vi "Create Menus.vi"(6 "menu options":cluster{"open":bool, "save":bool, "view":bool}={"open"=TRUE, "save"=FALSE, "view"=FALSE}, 8 "error in (no error)":errorcluster, 11 "Application Data in":T1) -> (0 "error out":errorcluster, 3 "Application Data out":T1)   [LabVIEW 2017, in "DSF Core.lvlib"]
uses:
  DSF Core.lvlib
  Application Data.ctl
  <vilib>/NI/Memory Manager/Classes/Pointer/Pointer.lvclass
  Classes/Framework/Framework.lvclass
  Buffer Reader/Buffer Data.ctl
  Classes/Buffer/Buffer.lvclass
  Classes/Status/Status.lvclass
  Typedefs/DSF Data Type.ctl
  Typedefs/DSF Engine Channel Configuration.ctl
  Typedefs/DSF Settings Info.ctl
  Typedefs/DSF Byte Order.ctl
  Typedefs/DSF Engine Framework Configuration.ctl
  Typedefs/DSF Engine Plugin Configuration.ctl
  Typedefs/DSF Timing Info.ctl
  Typedefs/DSF Engine Plugin Thread Configuration.ctl
  Typedefs/DSF Engine Transfer Group Configuration.ctl
  Typedefs/DSF Direction.ctl
  Typedefs/DSF Engine Transfer Configuration.ctl
  Typedefs/DSF Timeout Behavior.ctl
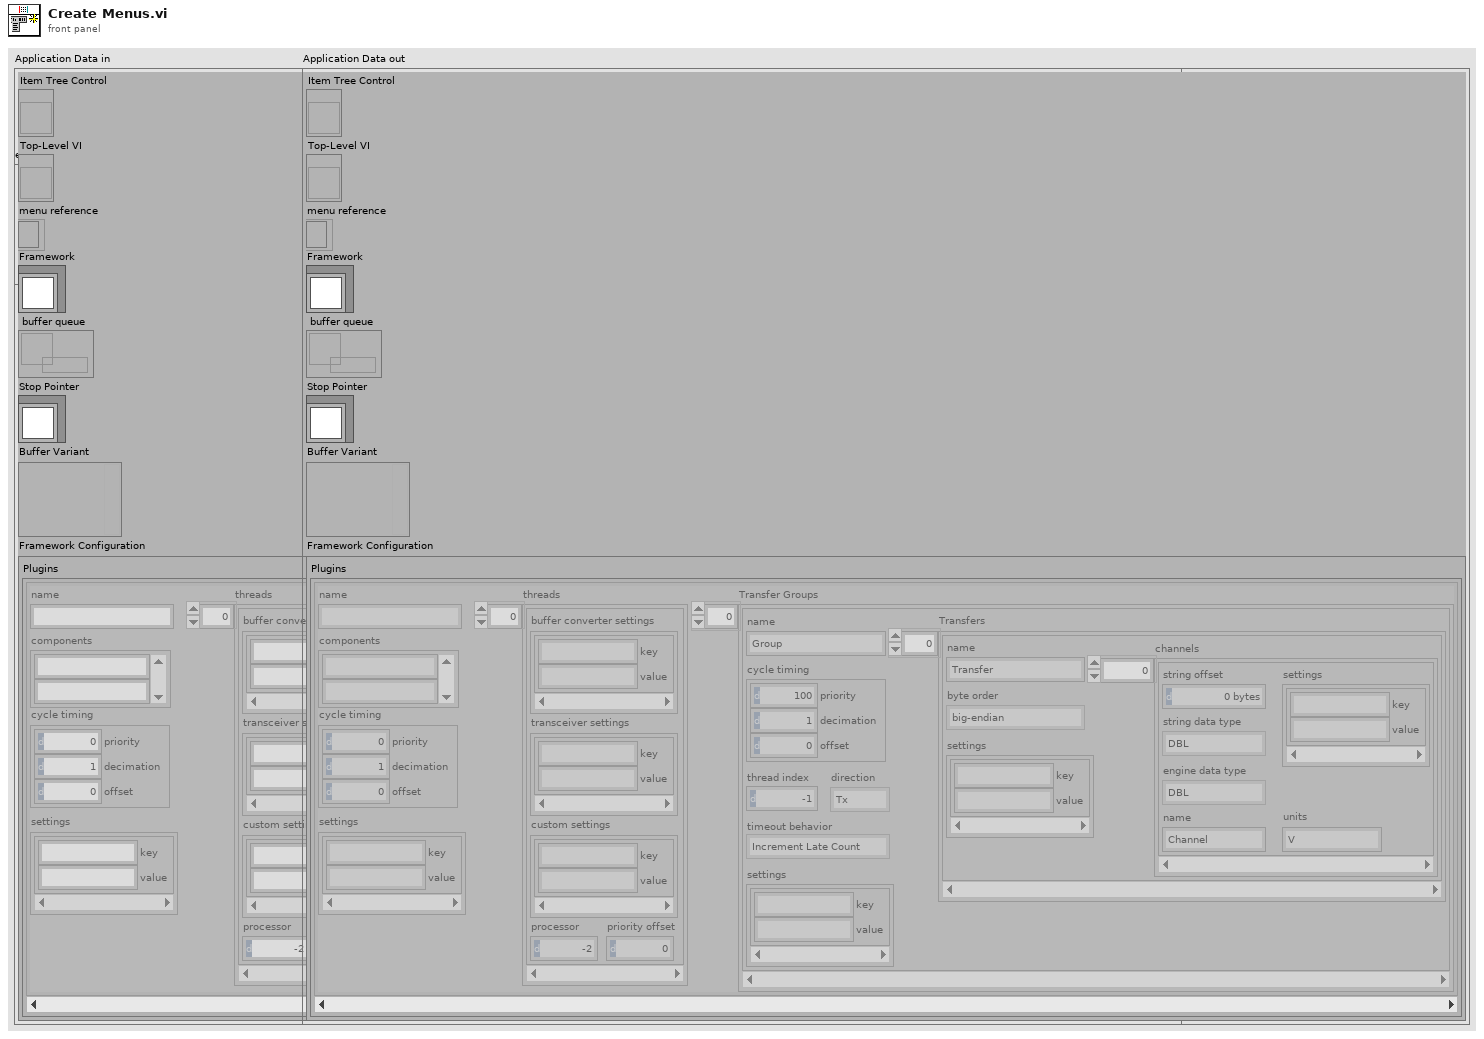
[diagram p1: front panel]
types:
  T1 = typedef "DSF Core.lvlib/Application Data.ctl" = cluster{"Item Tree Control":refnum<vi>, "Top-Level VI":refnum<vi>, "menu reference":refnum<k9>, "Framework":refnum<class "Framework.lvclass">, "buffer queue":refnum<queue>, "Stop Pointer":refnum<class "Pointer.lvclass">, "Buffer Variant":variant, "Framework Configuration":T2}
  T2 = typedef "DSF Core.lvlib/DSF Engine Framework Configuration.ctl" = cluster{"Plugins":T3[]}
  T3 = typedef "DSF Core.lvlib/DSF Engine Plugin Configuration.ctl" = cluster{"name":string, "components":string[], "cycle timing":T4, "threads":T5[], "Transfer Groups":T7[], "settings":T6}
  T4 = typedef "DSF Core.lvlib/DSF Timing Info.ctl" = cluster{"priority":u64, "decimation":u64, "offset":u64}
  T5 = typedef "DSF Core.lvlib/DSF Engine Plugin Thread Configuration.ctl" = cluster{"buffer converter settings":T6, "transceiver settings":T6, "custom settings":T6, "processor":i32, "priority offset":i16}
  T6 = typedef "DSF Core.lvlib/DSF Settings Info.ctl" = cluster{"key":string, "value":string}[]
  T7 = typedef "DSF Core.lvlib/DSF Engine Transfer Group Configuration.ctl" = cluster{"name":string, "direction":T8, "cycle timing":T4, "thread index":i32, "settings":T6, "Transfers":T9[], "timeout behavior":T13}
  T8 = typedef "DSF Core.lvlib/DSF Direction.ctl" = enum8{"Tx", "Rx"}
  T9 = typedef "DSF Core.lvlib/DSF Engine Transfer Configuration.ctl" = cluster{"name":string, "byte order":T10, "settings":T6, "channels":T11[]}
  T10 = typedef "DSF Core.lvlib/DSF Byte Order.ctl" = enum8{"big-endian", "little-endian"}
  T11 = typedef "DSF Core.lvlib/DSF Engine Channel Configuration.ctl" = cluster{"string offset":u64, "string data type":T12, "engine data type":T12, "name":string, "settings":T6, "units":string}
  T12 = typedef "DSF Core.lvlib/DSF Data Type.ctl" = enum8{"Bool", "SGL", "DBL", "I8", "I16", "I32", "I64", "U8", "U16", "U32", "U64"}
  T13 = typedef "DSF Core.lvlib/DSF Timeout Behavior.ctl" = enum8{"Increment Late Count", "Throw Error"}
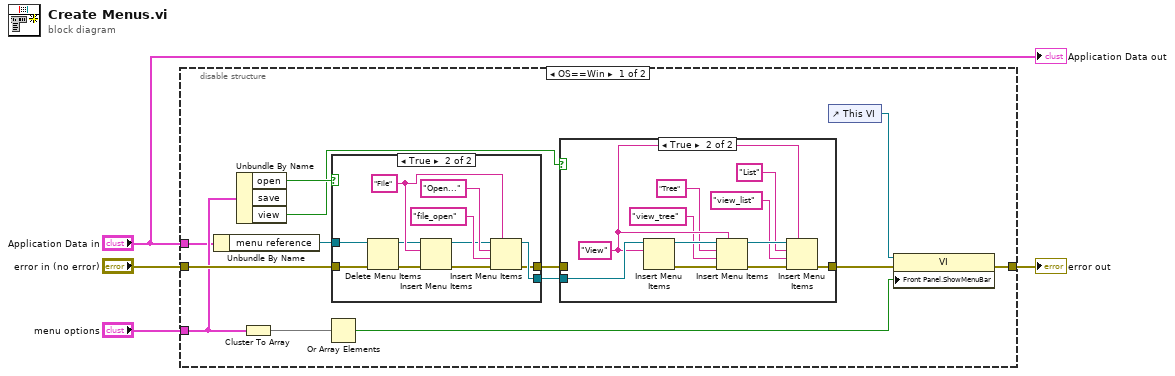
[diagram p0: block diagram]
diagram:
  n1 = disable-structure shown="OS==Win" {
    disable-tunnel: "error in (no error)" -> [w17 w43]
    disable-tunnel: "menu options" -> [w12 _]
    disable-tunnel: [w7 w43] -> w2
    disable-tunnel: "Application Data in" -> [w6 _]
    frame condition #0 (active) {
      n2 = Unbundle By Name(w6) -> ("menu reference"=w5:refnum<k9>)
      n3 = Unbundle By Name(w12) -> ("open"=w15:bool, "view"=w14:bool)  [unwired: 1 out]
      n4 = Cluster To Array(cluster=w12) -> (array=w11:bool[])
      n5 = Or Array Elements(Boolean array=w11) -> (logical OR=w9:bool)
      n6 = case shown="True" w15 {
        tunnel: w17 -> [w30 w42]
        tunnel: [w31 w40] -> w16
        tunnel: w5 -> [w31 w33]
        tunnel: [w30 w32] -> w13
        frame False {
        }
        frame True {
          w37 = "File" ("item names")
          n7 = Delete Menu Items(6:w42, 9:w33) -> (0:w41:errorcluster, 3:w34:refnum<k9>)  [unwired: 2 in]
          n8 = Insert Menu Items(6:w41, 8:w37, 9:w34) -> (0:w35:errorcluster, 3:w36:refnum<k9>)  [unwired: 3 in, 1 out]
          n9 = Insert Menu Items(5:w37, 6:w35, 7:"file_open" ("item tags"), 8:"Open..." ("item names"), 9:w36) -> (0:w32:errorcluster, 3:w40:refnum<k9>)  [unwired: 1 in, 1 out]
        }
      }
      n10 = case shown="True" w14 {
        tunnel: [w18 w29] -> w8
        tunnel: w16 -> [_ w28]
        tunnel: w13 -> [w18 _]
        frame False {
        }
        frame True {
          w26 = "View" ("item names")
          n11 = Insert Menu Items(8:w26, 9:w28) -> (0:w22:errorcluster, 3:w21:refnum<k9>)  [unwired: 4 in, 1 out]
          n12 = Insert Menu Items(5:w26, 6:w22, 7:"view_tree" ("item tags"), 8:"Tree" ("item names"), 9:w21) -> (0:w27:errorcluster, 3:w25:refnum<k9>)  [unwired: 1 in, 1 out]
          n13 = Insert Menu Items(5:w26, 6:w27, 7:"view_list" ("item tags"), 8:"List" ("item names"), 9:w25) -> (0:w29:errorcluster)  [unwired: 1 in, 2 out]
        }
      }
      n14 = control-ref of="This VI"() -> (w10:refnum<vi>)
      n15 = property class="VI"(reference=w10, error in=w8, "Front Panel.ShowMenuBar"=w9) -> (error out=w7:errorcluster)  [unwired: 1 out]
    }
    frame condition #1 {
    }
  }
  "error out" <- w2
  "Application Data out" <- "Application Data in"
